vi "CRYAPI LIST.vi"(0 "sAction":string="asada", 1 "WindowNumber":i32, 2 "List_In":cluster{"nID":i32, "pVIRef":refnum<vi>}[](array[cluster]), 3 "MousePos":T1) -> (7 "List_Out":cluster{"nID":i32, "pVIRef":refnum<vi>}[](array[cluster]), 8 "pVIRef_Out":refnum<vi>, 9 "nData_Out":i32, 10 "bResult":bool=TRUE)   [LabVIEW 2013]
uses:
  CRYMain Sub Window Global.vi
panel:
  out "Max":i32
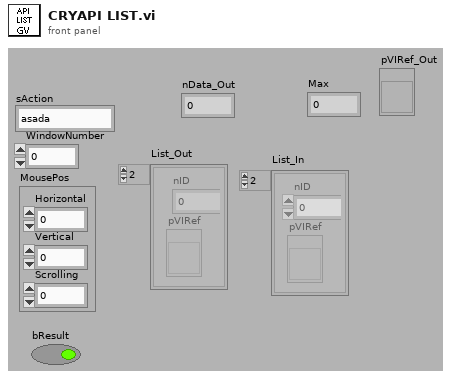
[diagram p1: front panel]
types:
  T1 = cluster{"Horizontal":i32, "Vertical":i32, "Scrolling":i32}
  T2 = enum32{"Invalid", "Standard", "Closed", "Hidden", "Minimized", "Maximized"}
  T3 = typedef "LVRectTypeDef.ctl" = cluster{"Left":i16, "Top":i16, "Right":i16, "Bottom":i16}
  T4 = cluster{"nID":i32[], "Frame":cluster{"nType":i32, "nParent":i32, "pVIW":refnum<vi>, "pSPW":refnum<vi>, "nTypeF":i32, "pVIF":refnum<vi>, "pSPF":refnum<vi>, "nIDSpliter":i32, "nProperty":i32, "Bound":T3, "nID":i32, "nData":i32, "sData":string, "pWVI":refnum<vi>, "sTitle":string, "cPages":cluster{"nPage":i32, "sTitle":string, "sIcon":string, "pVI":refnum<vi>, "nID":i32}[], "pTab":refnum<vi>, "nIDPages":i32[], "pSPT":refnum<vi>, "sTemp":string, "nDockID":i32, "nDockLR":i32, "sIcon":string}[]}
  T5 = cluster{"nType":i32, "nParent":i32, "pVIW":refnum<vi>, "pSPW":refnum<vi>, "nTypeF":i32, "pVIF":refnum<vi>, "pSPF":refnum<vi>, "nIDSpliter":i32, "nProperty":i32, "Bound":T3, "nID":i32, "nData":i32, "sData":string, "pWVI":refnum<vi>, "sTitle":string, "cPages":cluster{"nPage":i32, "sTitle":string, "sIcon":string, "pVI":refnum<vi>, "nID":i32}[], "pTab":refnum<vi>, "nIDPages":i32[], "pSPT":refnum<vi>, "sTemp":string, "nDockID":i32, "nDockLR":i32, "sIcon":string}[]
  T6 = cluster{"CLOSE_HIDE":i32, "CLOSE_CLOSE":i32, "DOCK_ENABLE":i32, "DOCK_DISABLE":i32, "FOCUS_SHOW":i32, "FOCUS_HIDE":i32}
  T7 = cluster{"nType":i32, "nParent":i32, "pVIW":refnum<vi>, "pSPW":refnum<vi>, "nTypeF":i32, "pVIF":refnum<vi>, "pSPF":refnum<vi>, "nIDSpliter":i32, "nProperty":i32, "Bound":T3, "nID":i32, "nData":i32, "sData":string, "pWVI":refnum<vi>, "sTitle":string, "cPages":cluster{"nPage":i32, "sTitle":string, "sIcon":string, "pVI":refnum<vi>, "nID":i32}[], "pTab":refnum<vi>, "nIDPages":i32[], "pSPT":refnum<vi>, "sTemp":string, "nDockID":i32, "nDockLR":i32, "sIcon":string}
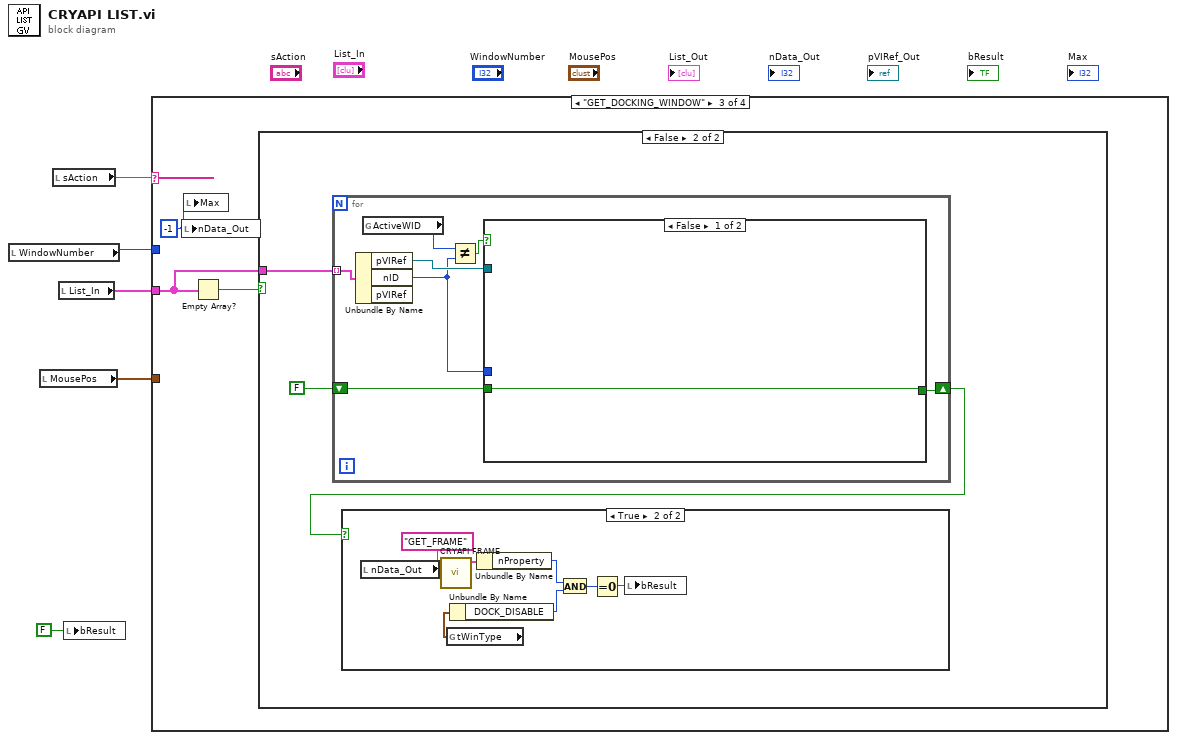
[diagram p0: block diagram]
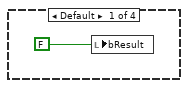
[diagram p2: hidden frame]
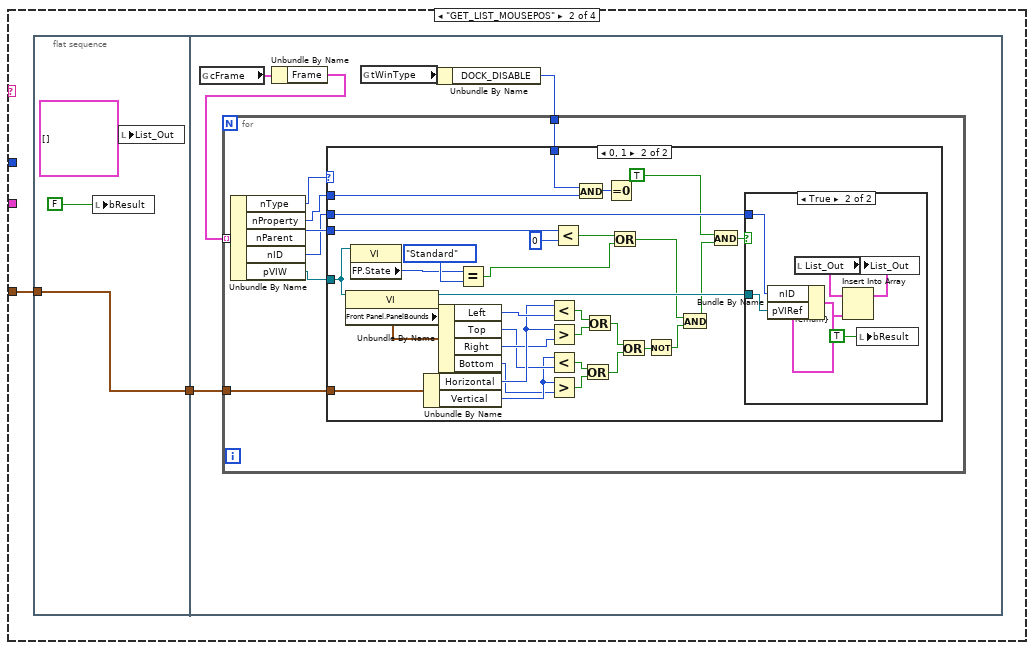
[diagram p3: hidden frame]
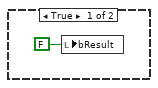
[diagram p6: hidden frame]
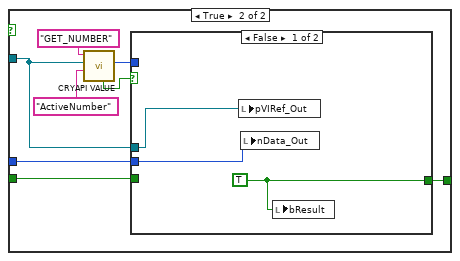
[diagram p8: hidden frame]
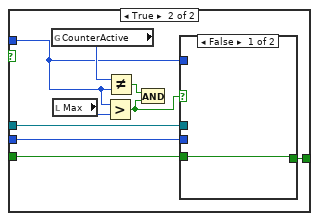
[diagram p9: hidden frame]
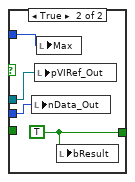
[diagram p10: hidden frame]
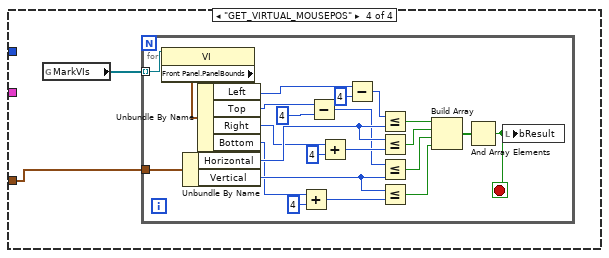
[diagram p11: hidden frame]
diagram:
  n1 = local read "WindowNumber"() -> (w4:i32)
  n2 = local read "MousePos"() -> (w3:T1)
  n3 = local read "sAction"() -> (w5:string)
  n4 = local read "List_In"() -> (w2:cluster{"nID":i32, "pVIRef":refnum<vi>}[])
  n5 = local write "bResult"(FALSE ("bResult")) -> ()
  n6 = case shown="\"GET_DOCKING_WINDOW\"" w5 {
    tunnel: w4 -> [_ _ _ _]
    tunnel: w3 -> [_ w8 _ w112]
    tunnel: w2 -> [_ _ w65 _]
    frame Default {
      n7 = local write "bResult"(FALSE ("bResult")) -> ()
    }
    frame "GET_LIST_MOUSEPOS" {
      n8 = flat-sequence {
        tunnel: w8 -> [w11]
        tunnel: [w11] -> w7
        tunnel: w7 -> [w16]
        frame #0 {
          n9 = local write "bResult"(FALSE ("bResult")) -> ()
          n10 = local write "List_Out"(cluster{"nID":i32, "pVIRef":refnum<vi>}[] [] ("List_Out")) -> ()
        }
        frame #1 {
          n11 = global read "CRYMain Sub Window Global.vi" "cFrame"() -> (w15:T4)
          n12 = Unbundle By Name(w15) -> ("Frame"=w14:T5)
          n13 = global read "CRYMain Sub Window Global.vi" "tWinType"() -> (w13:T6)
          n14 = Unbundle By Name(w13) -> ("DOCK_DISABLE"=w12:i32)
          n15 = for {
            tunnel: w16 -> [w24]
            tunnel: w14 -> [w23] mode=indexing
            tunnel: w12 -> [w17]
            n16 = Unbundle By Name(w23) -> ("nType"=w19:i32, "nProperty"=w18:i32, "nParent"=w22:i32, "nID"=w21:i32, "pVIW"=w20:refnum<vi>)
            n17 = case shown="0, 1" w19 {
              tunnel: w20 -> [_ w38]
              tunnel: w24 -> [_ w56]
              tunnel: w21 -> [_ w36]
              tunnel: w22 -> [_ w34]
              tunnel: w18 -> [_ w27]
              tunnel: w17 -> [_ w26]
              frame Default {
              }
              frame 0, 1 {
                n18 = property class="VI"(reference=w38) -> (reference out=w52:refnum<vi>, "Front Panel.PanelBounds"=w55:T3)  [unwired: 1 in, 1 out]
                n19 = property class="VI"(reference=w38) -> ("FP.State"=w53:T2)  [unwired: 1 in, 2 out]
                n20 = Unbundle By Name(w56) -> ("Horizontal"=w50:i32, "Vertical"=w47:i32)
                n21 = Unbundle By Name(w55) -> ("Left"=w51:i16, "Top"=w48:i16, "Right"=w49:i16, "Bottom"=w46:i16)
                n22 = Equal?(x=w53, y=T2."Standard" ("Front Panel Window:State")) -> (x = y?=w31:bool)
                n23 = Less?(x=w50, y=w51) -> (x < y?=w44:bool)
                n24 = Greater?(x=w50, y=w49) -> (0:w45:bool)
                n25 = Less?(x=w47, y=w48) -> (x < y?=w43:bool)
                n26 = Greater?(x=w47, y=w46) -> (0:w42:bool)
                n27 = Less?(x=w34, y=0) -> (x < y?=w32:bool)
                n28 = And(x=w26, y=w27) -> (x .and. y?=w30:i32)
                n29 = Or(x=w43, y=w42) -> (x .or. y?=w40:bool)
                n30 = Or(x=w44, y=w45) -> (x .or. y?=w41:bool)
                n31 = Equal To 0?(x=w30) -> ()  [unwired: 1 out]
                n32 = Or(x=w32, y=w31) -> (x .or. y?=w33:bool)
                n33 = Or(x=w41, y=w40) -> (x .or. y?=w39:bool)
                n34 = Not(x=w39) -> (.not. x?=w37:bool)
                n35 = And(x=w33, y=w37) -> (x .and. y?=w28:bool)
                n36 = And(x=TRUE, y=w28) -> (x .and. y?=w29:bool)
                n37 = case shown="True" w29 {
                  tunnel: w52 -> [_ w57]
                  tunnel: w36 -> [_ w58]
                  frame False {
                  }
                  frame True {
                    n38 = Bundle By Name(cluster=cluster{"nID":i32, "pVIRef":refnum<vi>} {"nID"=0, "pVIRef"=refnum} ("Cluster"), "nID"=w58, "pVIRef"=w57) -> (w59:cluster{"nID":i32, "pVIRef":refnum<vi>})
                    n39 = local read "List_Out"() -> (w63:cluster{"nID":i32, "pVIRef":refnum<vi>}[])
                    n40 = Insert Into Array(array=w63, new element=w59) -> (w62:cluster{"nID":i32, "pVIRef":refnum<vi>}[])  [unwired: 1 in]
                    n41 = local write "List_Out"(w62) -> ()
                    n42 = local write "bResult"(TRUE ("bResult")) -> ()
                  }
                }
              }
            }
          }
        }
      }
    }
    frame "GET_DOCKING_WINDOW" {
      w66 = -1 ("nData")
      n43 = local write "nData_Out"(w66) -> ()
      n44 = local write "Max"(w66) -> ()
      n45 = Empty Array?(array=w65) -> (empty?=w64:bool)
      n46 = case shown="False" w64 {
        tunnel: w65 -> [_ w70]
        frame True {
          n47 = local write "bResult"(FALSE ("bResult")) -> ()
        }
        frame False {
          n48 = for {
            tunnel: w70 -> [w83] mode=indexing
            shift-right: [w79] -> w68
            shift-left: FALSE ("bResult") -> [w80]
            n49 = Unbundle By Name(w83) -> ("pVIRef"=w82:refnum<vi>, "nID"=w81:i32)  [unwired: 1 out]
            n50 = global read "CRYMain Sub Window Global.vi" "ActiveWID"() -> (w84:i32)
            n51 = Not Equal?(x=w84, y=w81) -> (x != y?=w85:bool)
            n52 = case shown="False" w85 {
              tunnel: w82 -> [_ w94]
              tunnel: w81 -> [_ w90]
              tunnel: w80 -> [w86 w88]
              tunnel: [w86 w87] -> w79
              frame False {
              }
              frame True {
                n53 = call "CRYAPI VALUE.vi"("sControlName"="ActiveNumber", "pVIRef"=w94, "sAction"="GET_NUMBER") -> ("Numeric"=w91:i32, "bResult"=w89:bool)  [unwired: 2 in, 5 out]
                n54 = case shown="False" w89 {
                  tunnel: w91 -> [_ w103]
                  tunnel: w94 -> [w97 w102]
                  tunnel: w90 -> [w96 w101]
                  tunnel: w88 -> [_ w99]
                  tunnel: [w95 w98] -> w87
                  frame False {
                    w95 = TRUE ("bResult")
                    n55 = local write "pVIRef_Out"(w97) -> ()
                    n56 = local write "nData_Out"(w96) -> ()
                    n57 = local write "bResult"(w95) -> ()
                  }
                  frame True {
                    n58 = global read "CRYMain Sub Window Global.vi" "CounterActive"() -> (w106:i32)
                    n59 = local read "Max"() -> (w105:i32)
                    n60 = Greater?(x=w103, y=w105) -> (0:w100:bool)
                    n61 = Not Equal?(x=w106, y=w103) -> (x != y?=w104:bool)
                    n62 = And(x=w104, y=w100) -> ()  [unwired: 1 out]
                    n63 = case shown="False" w100 {
                      tunnel: w103 -> [_ w111]
                      tunnel: w102 -> [_ w110]
                      tunnel: w101 -> [_ w109]
                      tunnel: w99 -> [w107 _]
                      tunnel: [w107 w108] -> w98
                      frame False {
                      }
                      frame True {
                        w108 = TRUE ("bResult")
                        n64 = local write "nData_Out"(w109) -> ()
                        n65 = local write "pVIRef_Out"(w110) -> ()
                        n66 = local write "Max"(w111) -> ()
                        n67 = local write "bResult"(w108) -> ()
                      }
                    }
                  }
                }
              }
            }
          }
          n68 = case shown="True" w68 {
            frame False {
            }
            frame True {
              n69 = local read "nData_Out"() -> (w76:i32)
              n70 = call "CRYAPI FRAME.vi"("nData"=w76, "sAction"="GET_FRAME") -> ("tFrame_Out"=w75:T7)  [unwired: 4 in, 5 out]
              n71 = global read "CRYMain Sub Window Global.vi" "tWinType"() -> (w78:T6)
              n72 = Unbundle By Name(w78) -> ("DOCK_DISABLE"=w73:i32)
              n73 = Unbundle By Name(w75) -> ("nProperty"=w74:i32)
              n74 = And(x=w74, y=w73) -> (x .and. y?=w72:i32)
              n75 = Equal To 0?(x=w72) -> (x = 0?=w71:bool)
              n76 = local write "bResult"(w71) -> ()
            }
          }
        }
      }
    }
    frame "GET_VIRTUAL_MOUSEPOS" {
      n77 = global read "CRYMain Sub Window Global.vi" "MarkVIs"() -> (w113:refnum<vi>[])
      n78 = for {
        tunnel: w112 -> [w117]
        tunnel: w113 -> [w116] mode=indexing
        stop <- w115 stop-if-true
        n79 = property class="VI"(reference=w116) -> ("Front Panel.PanelBounds"=w134:T3)  [unwired: 1 in, 2 out]
        n80 = Unbundle By Name(w117) -> ("Horizontal"=w136:i32, "Vertical"=w135:i32)
        n81 = Unbundle By Name(w134) -> ("Left"=w121:i16, "Top"=w119:i16, "Right"=w123:i16, "Bottom"=w125:i16)
        n82 = Add(x=w125, y=4) -> (x+y=w124:i32)
        n83 = Subtract(x=w119, y=4) -> (x-y=w118:i32)
        n84 = Add(x=w123, y=4) -> (x+y=w122:i32)
        n85 = Subtract(x=w121, y=4) -> (x-y=w120:i32)
        n86 = Less Or Equal?(x=w120, y=w136) -> (x <= y?=w133:bool)
        n87 = Less Or Equal?(x=w136, y=w122) -> (x <= y?=w132:bool)
        n88 = Less Or Equal?(x=w118, y=w135) -> (x <= y?=w131:bool)
        n89 = Less Or Equal?(x=w135, y=w124) -> (x <= y?=w130:bool)
        n90 = Build Array(w133, w132, w131, w130) -> (w129:bool[])
        n91 = And Array Elements(Boolean array=w129) -> (logical AND=w115:bool)
        n92 = local write "bResult"(w115) -> ()
      }
    }
  }
